vi "writeSGLFIFO.vi"(8 "error in (no error)":errorcluster, 9 "Timeout":i32, 10 "Data":sgl[](array[numeric]), 11 "IWriteSGLFIFO in":refnum<class "IWriteSGLFIFO.lvclass">) -> (0 "error out":errorcluster, 2 "ElementsRemaining":u32, 3 "IWriteSGLFIFO out":refnum<class "IWriteSGLFIFO.lvclass">)   [LabVIEW 2016, in "RTFPGA.lvlib" / "IWriteSGLFIFO.lvclass"]
uses:
  IWriteSGLFIFO.lvclass
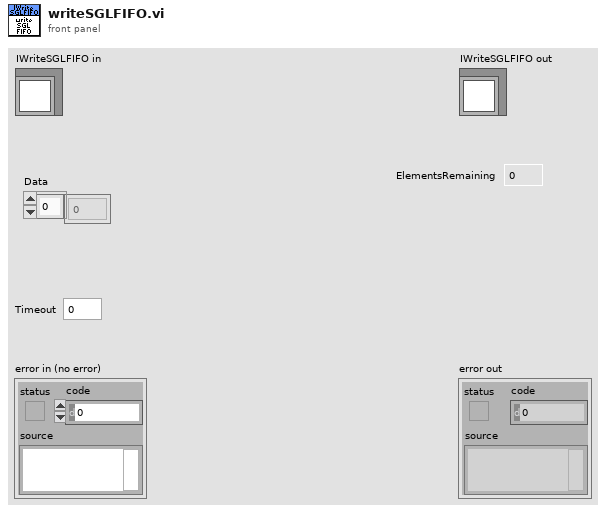
[diagram p1: front panel]
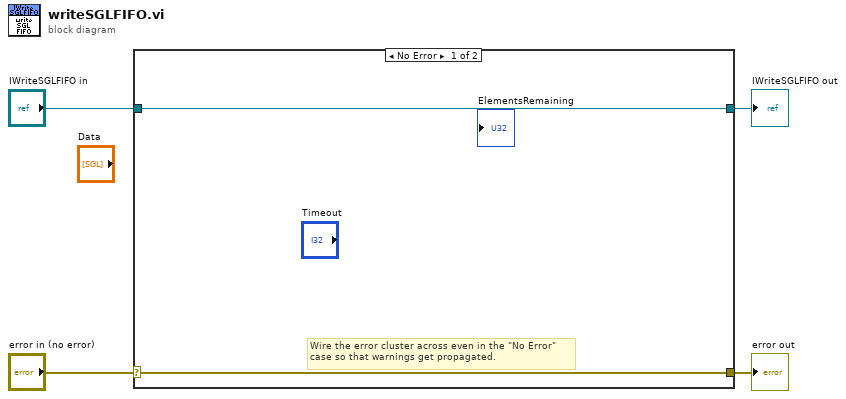
[diagram p0: block diagram]
diagram:
  n1 = case shown="No Error" "error in (no error)" {
    selector: "error in (no error)" -> [w5 w8]
    tunnel: [w5 w8] -> w3
    tunnel: [w6 w7] -> w1
    tunnel: "IWriteSGLFIFO in" -> [w6 w7]
    frame No Error {
      # "Wire the error cluster across even in the \"No Error\"\ncase so that warnings get propagated."
    }
    frame Error {
    }
  }
  "error out" <- w3
  "IWriteSGLFIFO out" <- w1
